vi "SetSizeAndOriginForMultiplot.vi"(4 "VerticalPosition":dbl, 5 "Height":dbl, 6 "LateralPosition":dbl, 7 "Width":dbl, 8 "ClearLabels?":bool, 9 "PlotLocationDescription":string="Top-left plot", 11 "gnuplotIn":string) -> (3 "gnuplotOut":string)   [LabVIEW 2013]
panel:
  out "resulting string":string
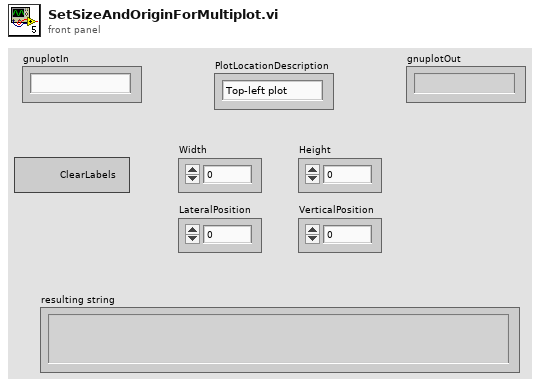
[diagram p1: front panel]
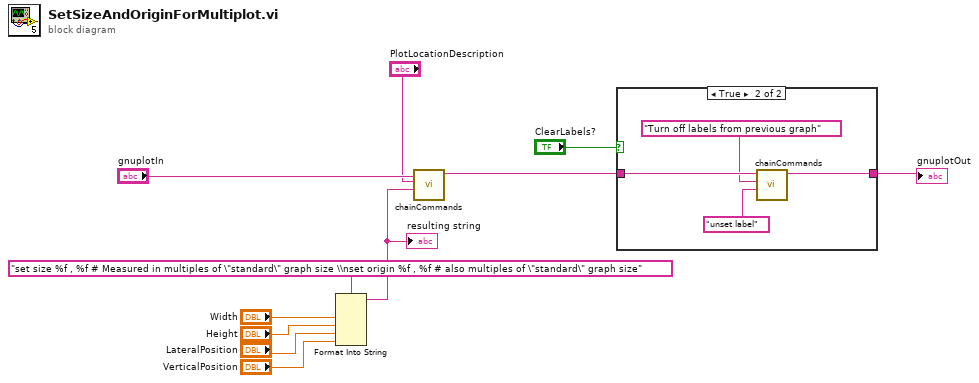
[diagram p0: block diagram]
diagram:
  n1 = Format Into String(format string="set size %f , %f # Measured in multiples of \"standard\" graph size \\nset origin %f , %f # also multiples of \"standard\" graph size", "Width", "Height", "LateralPosition", "VerticalPosition") -> (resulting string=w4:string)  [unwired: 2 in, 1 out]
  "resulting string" <- w4
  n2 = call "chainCommands.vi"("Command"=w4, "Comments"="PlotLocationDescription", "StringIn"="gnuplotIn") -> ("StringOut"=w3:string)  [unwired: 8 in]
  n3 = case shown="True" "ClearLabels?" {
    tunnel: w3 -> [w12 w16]
    tunnel: [w12 w15] -> w2
    frame False {
    }
    frame True {
      n4 = call "chainCommands.vi"("Command"="unset label", "Comments"="Turn off labels from previous graph", "StringIn"=w16) -> ("StringOut"=w15:string)  [unwired: 8 in]
    }
  }
  "gnuplotOut" <- w2
